vi "image navigation.vi"() -> ()   [LabVIEW 2009]
uses:
  <vilib>/picture/picture.llb/Draw 4-Bit Pixmap.vi
panel:
  out "time elapsed":u32
  out "x > 0?":bool[](array[boolean])
  in  "weighting":dbl[](array[numeric])
  in  "reset":bool
  in  "mouse?":bool
  out "color":bool[](array[boolean])
  out "direction":dbl(knob) scale=-3.141592653589793..3.141592653589793 scale format="%#.1f"
  in  "Path":path
  in  "speed":u8
  out "current point":cluster{"x":i16, "y":i16}
  in  "initial point":cluster{"x":i16, "y":i16}
  out "new picture":picture
  in  "stop":bool
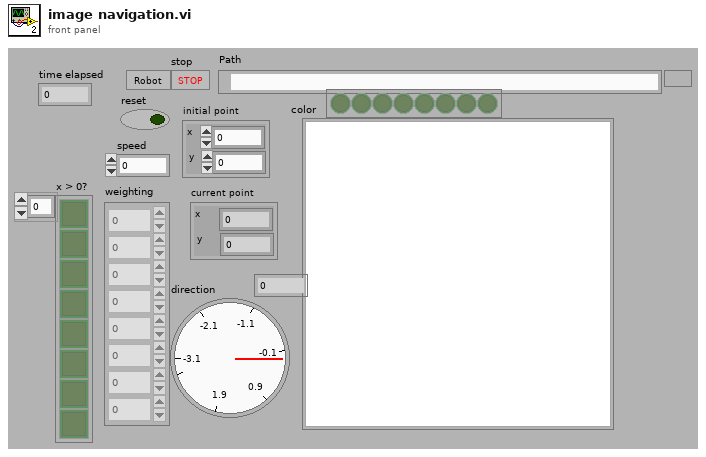
[diagram p1: front panel]
types:
  T1 = cluster{"spacing":i16, "radius":u16, "angle":dbl}[]
  T2 = typedef "imagedata.ctl" = cluster{"image type":i32, "image depth":i32, "image":u8[], "mask":u8[], "colors":u32[], "Rectangle":cluster{"left":i16, "top":i16, "right":i16, "bottom":i16}}
  T3 = cluster{"point":cluster{"x":i16, "y":i16}, "distance":u16, "theta":dbl}[]
  T4 = typedef "LVMouseTypeDef.ctl" = cluster{"Mouse Position":cluster{"X":i32, "Y":i32}, "Mouse Modifiers":cluster{"Button Down":bool, "Shift Mod":bool, "Menu Mod":bool, "Option Mod":bool}}
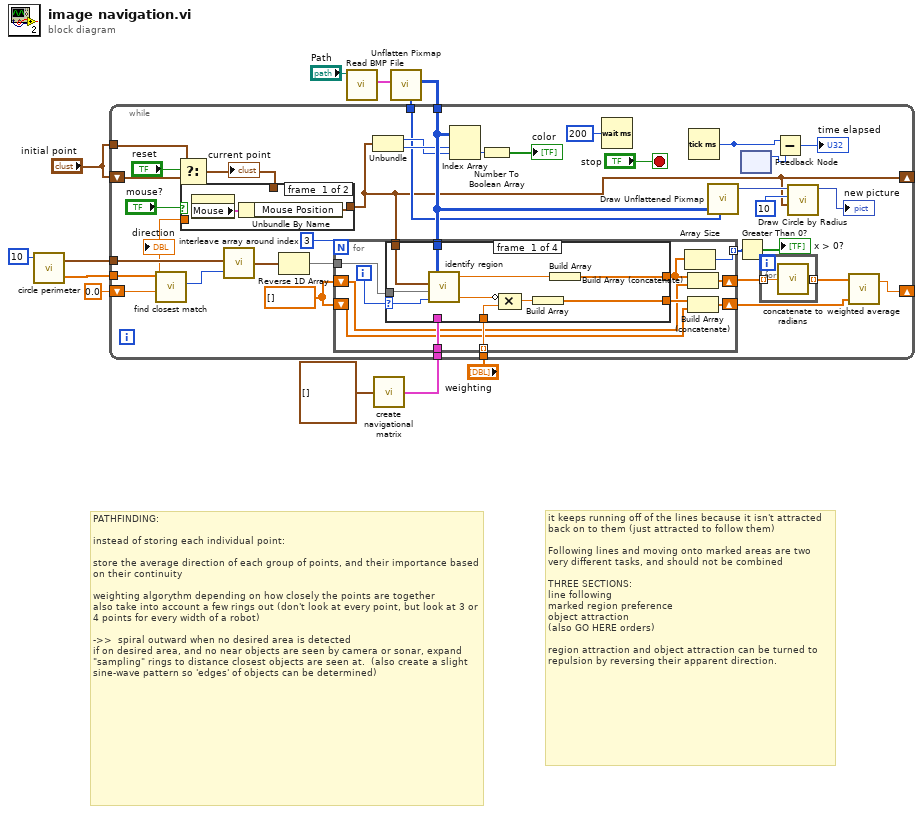
[diagram p0: block diagram]
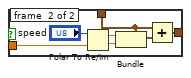
[diagram p2: hidden frame]
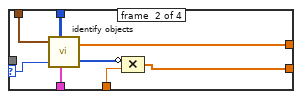
[diagram p3: hidden frame]
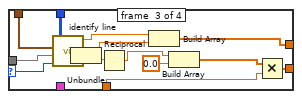
[diagram p4: hidden frame]
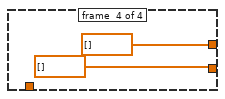
[diagram p5: hidden frame]
diagram:
  # "it keeps running off of the lines because it isn't attracted back on to them (just attracted to follow them)\n\nFollowing lines and moving onto marked areas are two very different tasks, and should not be combined\n\nTHREE SECTIONS:\nline following\nmarked region preference\nobject attraction\n(also GO HERE orders)\n\nregion attraction and object attraction can be turned to repulsion by reversing their apparent direction."
  # "PATHFINDING:\n\ninstead of storing each individual point:\n\nstore the average direction of each group of points, and their importance based on their continuity\n\nweighting algorythm depending on how closely the points are together\nalso take into account a few rings out (don't look at every point, but look at 3 or 4 points for every width of a robot)\n\n->>  spiral outward when no desired area is detected\nif on desired area, and no near objects are seen by camera or sonar, expand \"sampling\" rings to distance closest objects are seen at.  (also create a slight sine-wave pattern so 'edges' of objects can be determined)"
  n1 = call "circle perimeter.vi"("radius"=10) -> ("theta"=w9:dbl[], "points along perimeter"=w10:cluster{"x":i16, "y":i16}[])  [unwired: 3 in]
  n2 = call <vilib>:"Read BMP File.vi"("path to BMP file"="Path") -> ("image data"=w12:T2)  [unwired: 8 in, 2 out]
  n3 = call "create navigational matrix.vi"("parameters"=T1 []) -> ("Array"=w3:T3)
  n4 = call <vilib>:"Unflatten Pixmap.vi"("image data"=w12) -> ("8-bit pixmap"=w6:u8[][], "colors"=w5:u32[])  [unwired: 4 in, 5 out]
  n5 = while {
    tunnel: w10 -> [w44]
    tunnel: w6 -> [w40]
    shift-right: [w22] -> _
    shift-left: "initial point" -> [w34]
    tunnel: w9 -> [w45]
    shift-right: [w25] -> _
    shift-left: 0.0 -> [w27]
    tunnel: "initial point" -> [w33]
    tunnel: w5 -> [w30]
    tunnel: w3 -> [w26]
    tunnel: "weighting" -> [w24]
    stop <- "stop" stop-if-true
    w18 = dbl[] []
    n6 = call "find closest match.vi"("target element"=w27, "Array"=w45) -> ("index"=w43:i32)  [unwired: 2 in, 3 out]
    n7 = Select(t=w33, s="reset", f=w34) -> (s? t:f=w35:cluster{"X":i32, "Y":i32})
    "current point" <- w35
    n8 = case shown="True" "mouse?" {
      tunnel: w35 -> [_ w55]
      tunnel: w27 -> [_ w54]
      tunnel: [w51 w53] -> w22
      frame #0 {
        n9 = property on="new picture" class="Pict"() -> ("Mouse"=w52:T4)  [unwired: 2 in, 2 out]
        n10 = Unbundle By Name(w52) -> ("Mouse Position"=w51:cluster{"X":i32, "Y":i32})
      }
      frame #1 {
        n11 = Polar To Re/Im(2:w54, 3:"speed") -> (0:w58:dbl, 1:w59:dbl)
        n12 = Bundle(cluster=w55, "X"=w59, "Y"=w58) -> (w57:cluster{"X":i32, "Y":i32})
        n13 = Add(x=w55, y=w57) -> (x+y=w53:cluster{"X":i32, "Y":i32})
      }
    }
    n14 = call "interleave array around index.vi"("index"=w43, "Array in"=w44) -> ("Array out"=w42:cluster{"x":i16, "y":i16}[])
    n15 = Reverse 1D Array(array=w42) -> (reversed array=w29:cluster{"x":i16, "y":i16}[])
    n16 = for {
      N: 3 -> [_]
      tunnel: w40 -> [w69]
      tunnel: w22 -> [w70]
      tunnel: w29 -> [w72]
      tunnel: w26 -> [w71]
      tunnel: w24 -> [w68] mode=indexing
      shift-right: [w67] -> w20
      shift-left: w18 -> [w63]
      shift-right: [w66] -> w23
      shift-left: w18 -> [w64]
      tunnel: [w60] -> _ mode=indexing
      tunnel: [w60] -> w17 mode=indexing
      i -> [w62]
      n17 = case shown="0.." w62 {
        selector: w62 -> [w80 w88 w102 _]
        tunnel: w72 -> [w81 _ w103 _]
        tunnel: w71 -> [_ w87 _ _]
        tunnel: w70 -> [w82 w89 w104 _]
        tunnel: w69 -> [w79 w90 w101 _]
        tunnel: w68 -> [w77 w84 w94 _]
        tunnel: [w75 w83 w95 dbl[] []] -> w65
        tunnel: [w74 w86 w93 dbl[] [] ("direction")] -> w61
        frame #0 {
          n18 = call "identify region.vi"("index"=w80, "points"=w81, "location"=w82, "8-bit pixmap"=w79) -> ("distance"=w78:dbl, "direction"=w73:dbl)  [unwired: 1 in]
          n19 = Compound Arithmetic op=MULTIPLY(invert w78, w77) -> (w76:dbl)
          n20 = Build Array(w76) -> (w75:dbl[])
          n21 = Build Array(w73) -> (w74:dbl[])
        }
        frame #1 {
          n22 = call "identify objects.vi"("location"=w89, "8-bit pixmap"=w90, "index"=w88, "navigational matrix"=w87) -> ("direction"=w86:dbl[], "distance"=w85:u16[])  [unwired: 1 in]
          n23 = Compound Arithmetic op=MULTIPLY(invert w85, w84) -> (w83:dbl[])
        }
        frame #2 {
          n24 = call "identify line.vi"("index"=w102, "points"=w103, "location"=w104, "8-bit pixmap"=w101) -> ("relative to location"=w99:cluster{"direction":dbl, "distance":dbl}, "direction"=w100:dbl)  [unwired: 1 in]
          n25 = Unbundle(w99) -> ("direction"=w98:dbl, "distance"=w97:dbl)
          n26 = Reciprocal(x=w97) -> (1/x=w96:dbl)
          n27 = Build Array(w100, w98) -> (w93:dbl[])
          n28 = Build Array(w96, 0.0 ("element")) -> (w91:dbl[])
          n29 = Multiply(x=w91, y=w94) -> (x*y=w95:dbl[])
        }
        frame #3 {
        }
      }
      n30 = Array Size(array=w61) -> (size(s)=w60:i32)
      n31 = Build Array (concatenate)(w61, w63) -> (w67:dbl[])
      n32 = Build Array (concatenate)(w65, w64) -> (w66:dbl[])
    }
    n33 = Unbundle(w22) -> ("X"=w36:i32, "Y"=w37:i32)
    n34 = Index Array(array=w40, index (row)=w37, index (col)=w36) -> (element=w39:u8)
    n35 = Number To Boolean Array(number=w39) -> (Boolean array=→"color":bool[])
    n36 = Wait (ms)(milliseconds to wait=u32 200) -> ()  [unwired: 1 out]
    n37 = Tick Count (ms)() -> (millisecond timer value=w14:u32)
    n38 = call-poly <vilib>:"Draw Unflattened Pixmap.vi"("data"=w40, "color table"=w30) -> ("new picture"=w41:picture)  [unwired: 7 in]
    n39 = Greater Than 0?(x=w17) -> (x > 0?=→"x > 0?":bool[])
    n40 = feedback #1() -> (w15:u32)  [unwired: 1 in]
    n41 = for {
      tunnel: w20 -> [w50] mode=indexing
      tunnel: [w49] -> w19 mode=indexing
      n42 = call "concatenate to radians.vi"("value"=w50) -> ("concatenated value"=w49:dbl)
    }
    n43 = Subtract(x=w14, y=w15) -> (x-y=→"time elapsed":u32)
    n44 = call <vilib>:"Draw Circle by Radius.vi"("pixel center"=w22, "radius"=i16 10, "picture"=w41) -> ("new picture"=→"new picture":picture)  [unwired: 8 in]
    n45 = call "weighted average.vi"("weighting"=w23, "elements"=w19) -> ("average"=w25:dbl)  [unwired: 2 in, 1 out]
    "direction" <- w27
  }
